vi "Wire FP Controls to Bundler.vi"(8 "error in (no error)":errorcluster, 10 "Controls":refnum<vi>[](array[refnum]), 11 "vi reference in":refnum<vi>) -> (0 "error out":errorcluster, 3 "vi reference out":refnum<vi>)   [LabVIEW 2020, in "Message Maker.lvlib"]
uses:
  Message Maker.lvlib
  <vilib>/Utility/traverseref.llb/TRef TravTarget.ctl
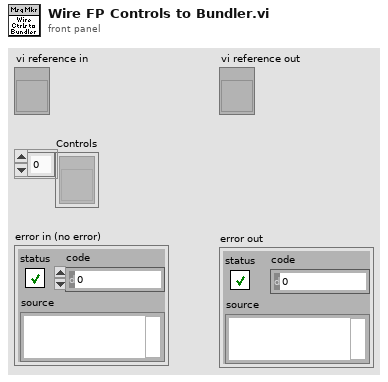
[diagram p1: front panel]
types:
  T1 = typedef "TRef TravTarget.ctl" = enum16{"FP", "BD", "Other"}
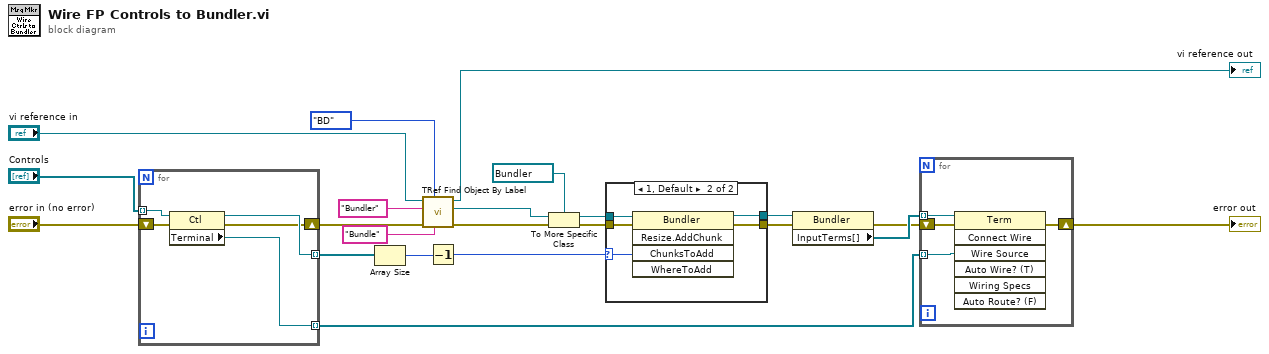
[diagram p0: block diagram]
diagram:
  n1 = for {
    tunnel: [w27] -> w20 mode=indexing
    tunnel: "Controls" -> [w26] mode=indexing
    shift-right: [w24] -> w5
    shift-left: "error in (no error)" -> [w25]
    tunnel: [w23] -> w22 mode=indexing
    n2 = property class="Ctl"(reference=w26, error in=w25) -> (reference out=w27:refnum<vi>, error out=w24:errorcluster, "Terminal"=w23:refnum<vi>)
  }
  n3 = Array Size(array=w20) -> (size(s)=w14:i32)
  n4 = call <vilib>:"TRef Find Object By Label.vi"("Label"="Bundle", "Traverse Target"=TRef_TravTarget."BD", "error in (no error)"=w5, "Class Name"="Bundler", "VI Ref"="vi reference in") -> ("error out"=w3:errorcluster, "Found Obj Ref"=w4:refnum<vi>, "dup VI Ref"=→"vi reference out":refnum<vi>)  [unwired: 3 in, 1 out]
  n5 = Decrement(x=w14) -> (x-1=w10:i32)
  n6 = To More Specific Class(target class=refnum<vi> refnum ("reference"), reference=w4, error in=w3) -> (specific class reference=w12:refnum<vi>, error out=w13:errorcluster)
  n7 = case shown="1, Default" w10 {
    selector: w10 -> [_ w30]
    tunnel: [w28 w34] -> w16
    tunnel: [w29 w33] -> w15
    tunnel: w13 -> [w28 w32]
    tunnel: w12 -> [w29 w31]
    frame ..0 {
    }
    frame 1, Default {
      n8 = invoke class="Bundler" method="Resize.AddChunk"(reference=w31, error in=w32, "ChunksToAdd"=w30) -> (reference out=w33:refnum<vi>, error out=w34:errorcluster)  [unwired: 2 in, 3 out]
    }
  }
  n9 = property class="Bundler"(reference=w15, error in=w16) -> (error out=w19:errorcluster, "InputTerms[]"=w21:refnum<vi>[])  [unwired: 1 out]
  n10 = for {
    tunnel: w22 -> [w36] mode=indexing
    shift-right: [w35] -> w9
    shift-left: w19 -> [w37]
    tunnel: w21 -> [w38] mode=indexing
    n11 = invoke class="Term" method="Connect Wire"(reference=w38, error in=w37, "Wire Source"=w36) -> (error out=w35:errorcluster)  [unwired: 4 in, 6 out]
  }
  "error out" <- w9
